vi "Keithley_Control.vi"(0 "VISA resource name":refnum<visa-resource-name>, 1 "Set Value":bool, 5 "Source Mode  (0: Voltage)":u16(ring) items=["Voltage", "Current"], 7 "Output Level (0)":dbl, 9 "Compliance  Level (0.1)":dbl=0.1, 11 "error in (no error)":errorcluster) -> (4 "Voltage":sgl, 6 "Current":sgl, 15 "error out":errorcluster)   [LabVIEW 2019]
doc: "This example shows how to configure a measurement and take a reading."
uses:
  Keithley/Keithley 24XX/Public/Data/Read (Single Point).vi
  Keithley/Keithley 24XX/Keithley 24XX.lvlib
panel:
  in  "stop":bool
  in  "Enable Resistance Auto Range (T:Enable)":bool=TRUE
  in  "Enable Current Auto Range (T:Enable)":bool=TRUE
  in  "Enable Voltage Auto Range (T:Enable)":bool=TRUE
  in  "Resistance Manual Range (1.0)":dbl=1.0
  in  "Current Manual Range (1.0)":dbl=1.0
  in  "Voltage Manual Range (1.0)":dbl=1.0
  out "Resistance":sgl
  in  "Serial Configuration":T1={"Baud Rate"=9600, "Parity"=0, "Data Bits"=8, "Stop Bits"=10, "Flow Control"=0} {"Flow Control" items=["None", "XON/XOFF", "RTS/CTS", "XON/XOFF & RTS/CTS", "DTR/DSR", "XON/XOFF & DTR/DSR"]; "Stop Bits" items=["1.0"=10, "1.5"=15, "2.0"=20]; "Data Bits" items=["7"=7, "8"=8]; "Parity" items=["None", "Odd", "Even", "Mark", "Space"]; "Baud Rate" items=["300"=300, "600"=600, "1200"=1200, "2400"=2400, "4800"=4800, "9600"=9600, "19200"=19200]}
  # "Combo 1"
  # "(c) 2006 - 2015 National Instruments.  ALL RIGHTS RESERVED."
  # "Source Settings"
  # "Voltage Range Settings"
  # "Current Range Settings"
  # "Resistance Range Settings"
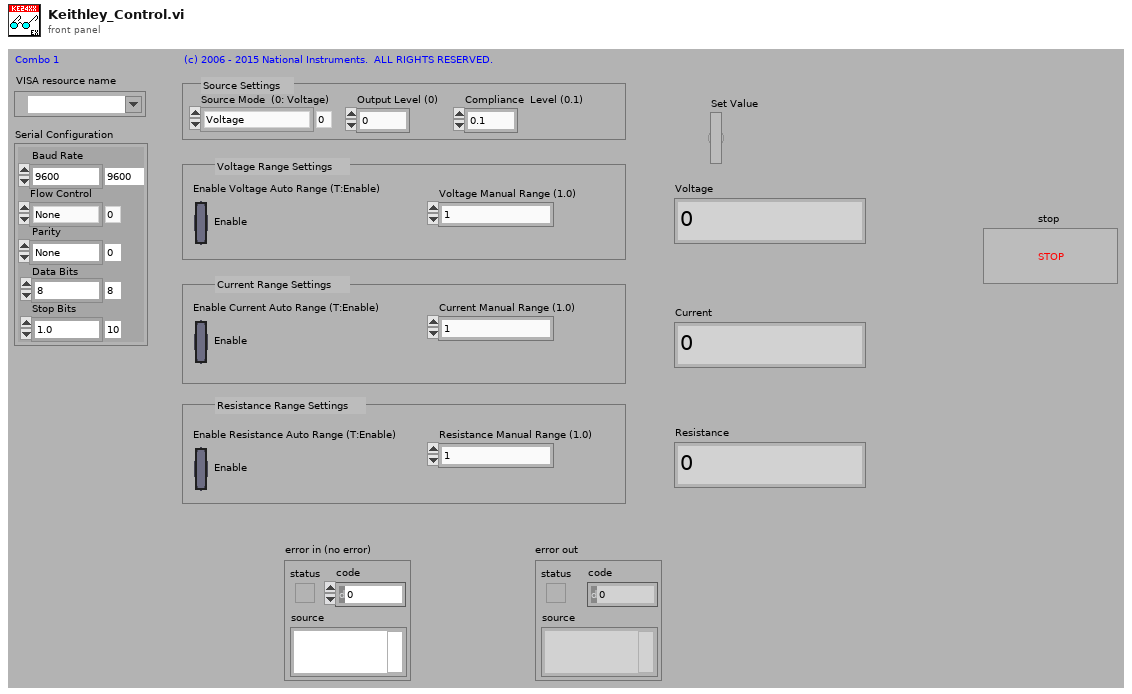
[diagram p1: front panel]
types:
  T1 = cluster{"Baud Rate":u32, "Parity":u16, "Data Bits":u16, "Stop Bits":u16, "Flow Control":u16}
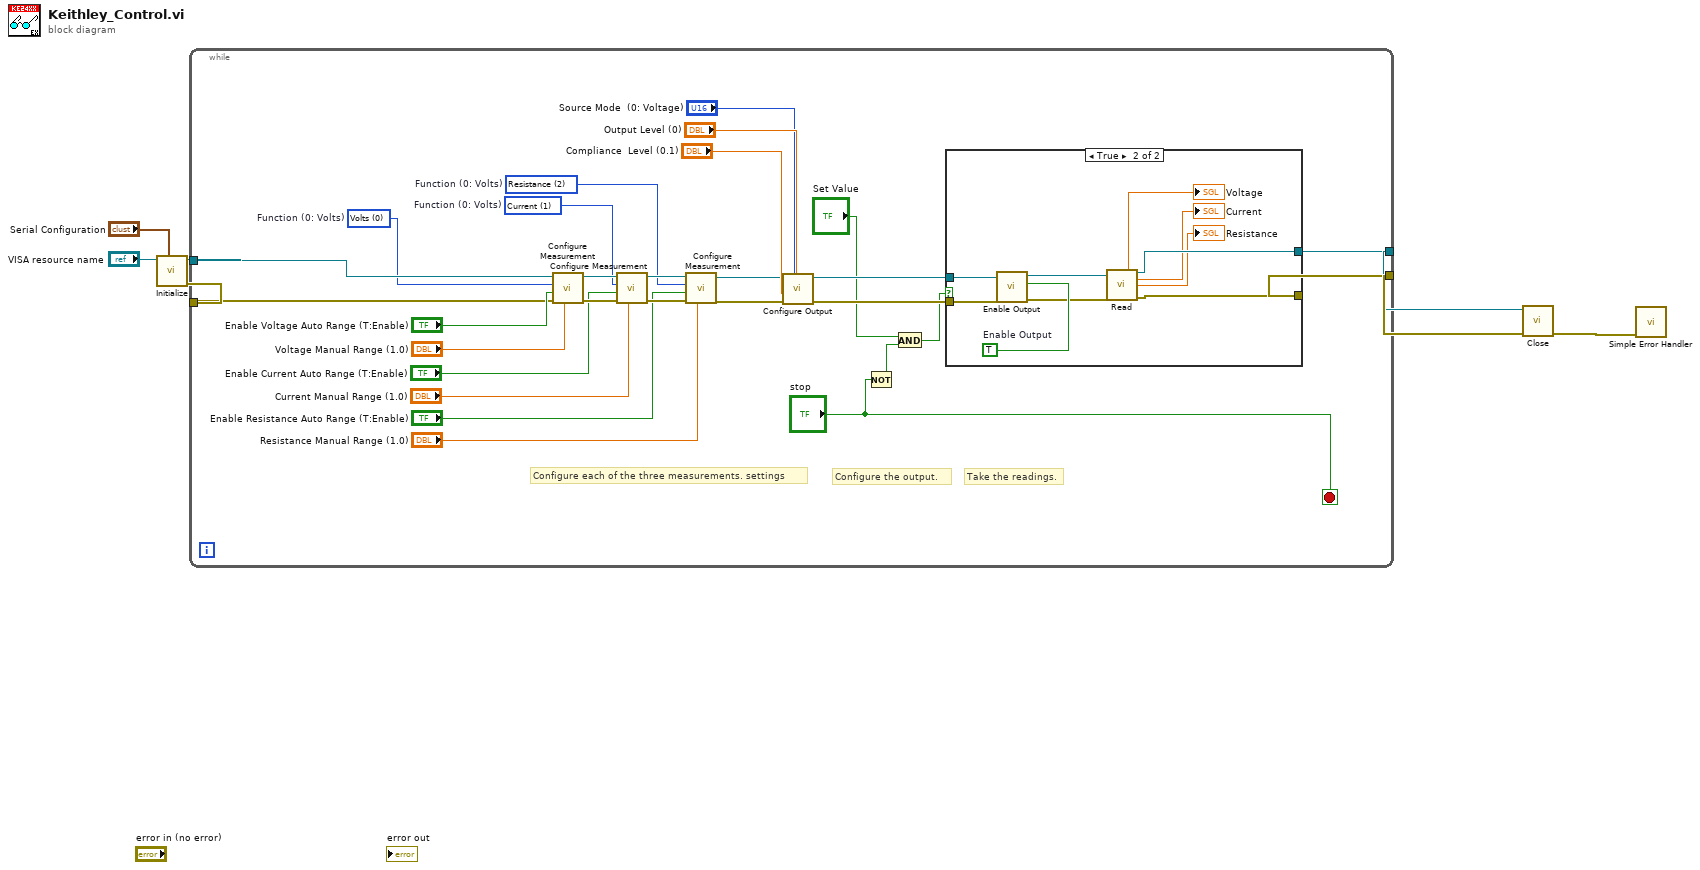
[diagram p0: block diagram]
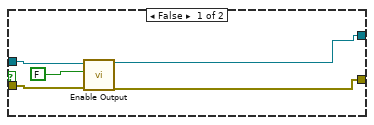
[diagram p2: hidden frame]
diagram:
  n1 = call "Initialize.vi"("Serial Configuration"="Serial Configuration", "VISA resource name"="VISA resource name") -> ("error out"=w5:errorcluster, "VISA resource name out"=w4:refnum<visa-resource-name>)  [unwired: 8 in]
  n2 = while {
    tunnel: w5 -> [w16]
    tunnel: w4 -> [w15]
    tunnel: [w12] -> w2
    tunnel: [w13] -> w1
    stop <- "stop" stop-if-true
    w14 = u16 0 items=["Volts", "Current", "Resistance"]  # Function (0: Volts)
    w30 = u16 2 items=["Volts", "Current", "Resistance"]  # Function (0: Volts)
    w31 = u16 1 items=["Volts", "Current", "Resistance"]  # Function (0: Volts)
    # "Take the readings."
    # "Configure the output."
    # "Configure each of the three measurements. settings"
    n3 = call "Configure Measurement.vi"("Manual Range (1.0)"="Voltage Manual Range (1.0)", "error in (no error)"=w16, "Enable Auto Range (T:Enable)"="Enable Voltage Auto Range (T:Enable)", "Function (0: Volts)"=w14, "VISA resource name"=w15) -> ("error out"=w34:errorcluster, "VISA resource name out"=w35:refnum<visa-resource-name>)  [unwired: 5 in]
    n4 = call "Configure Measurement.vi"("Manual Range (1.0)"="Current Manual Range (1.0)", "error in (no error)"=w34, "Enable Auto Range (T:Enable)"="Enable Current Auto Range (T:Enable)", "Function (0: Volts)"=w31, "VISA resource name"=w35) -> ("error out"=w33:errorcluster, "VISA resource name out"=w32:refnum<visa-resource-name>)  [unwired: 5 in]
    n5 = call "Configure Measurement.vi"("Manual Range (1.0)"="Resistance Manual Range (1.0)", "error in (no error)"=w33, "Enable Auto Range (T:Enable)"="Enable Resistance Auto Range (T:Enable)", "Function (0: Volts)"=w30, "VISA resource name"=w32) -> ("error out"=w19:errorcluster, "VISA resource name out"=w18:refnum<visa-resource-name>)  [unwired: 5 in]
    n6 = call "Configure Output.vi"("Source Mode  (0: Voltage)"="Source Mode  (0: Voltage)", "error in (no error)"=w19, "Compliance  Level (0.1)"="Compliance  Level (0.1)", "Output Level (0)"="Output Level (0)", "VISA resource name"=w18) -> ("error out"=w20:errorcluster, "VISA resource name out"=w21:refnum<visa-resource-name>)  [unwired: 5 in]
    n7 = Not(x="stop") -> (.not. x?=w10:bool)
    n8 = And(x="Set Value", y=w10) -> (x .and. y?=w8:bool)
    n9 = case shown="True" w8 {
      tunnel: w21 -> [w40 w50]
      tunnel: w20 -> [w39 w49]
      tunnel: [w37 w45] -> w13
      tunnel: [w36 w44] -> w12
      frame False {
        n10 = call "Enable Output.vi"("error in (no error)"=w39, "Enable Output (T: Enable)"=FALSE, "VISA resource name"=w40) -> ("error out"=w36:errorcluster, "VISA resource name out"=w37:refnum<visa-resource-name>)  [unwired: 7 in]
      }
      frame True {
        w48 = TRUE  # Enable Output
        n11 = call "Enable Output.vi"("error in (no error)"=w49, "Enable Output (T: Enable)"=w48, "VISA resource name"=w50) -> ("error out"=w46:errorcluster, "VISA resource name out"=w47:refnum<visa-resource-name>)  [unwired: 7 in]
        n12 = call-poly "Read.vi"("VISA resource name"=w47, "error in (no error)"=w46) -> ("Voltage"=→"Voltage":sgl, "VISA resource name out"=w45:refnum<visa-resource-name>, "Current"=→"Current":sgl, "Resistance"=→"Resistance":sgl, "error out"=w44:errorcluster)  [unwired: 7 in, 2 out]
      }
    }
  }
  n13 = call "Close.vi"("error in (no error)"=w2, "VISA resource name"=w1) -> ("error out"=w3:errorcluster)  [unwired: 9 in]
  n14 = call <vilib>:"Simple Error Handler.vi"("error in (no error)"=w3) -> ()  [unwired: 4 in, 5 out]
